vi "test_firmware.vi"() -> ()   [LabVIEW 2025]
panel:
  out "ESP32 Listo":bool
  in  "Close":bool
  out "error out":errorcluster
  in  "stop":bool
  in  "Puerto COM":refnum<visa-resource-name>
  # "Este VI es para comprobar si el firmware fue subido correctamente\nSelecciona el puerto en donde este conectada la ESP32 \nLuego presiona el boton RST de la ESP32\nEspera unos segundos a que este cargue y si todo fue subido correctamente el led se va a encender y la ESP32 ya esta lista para usarse"
  # "Prueba de Firmware"
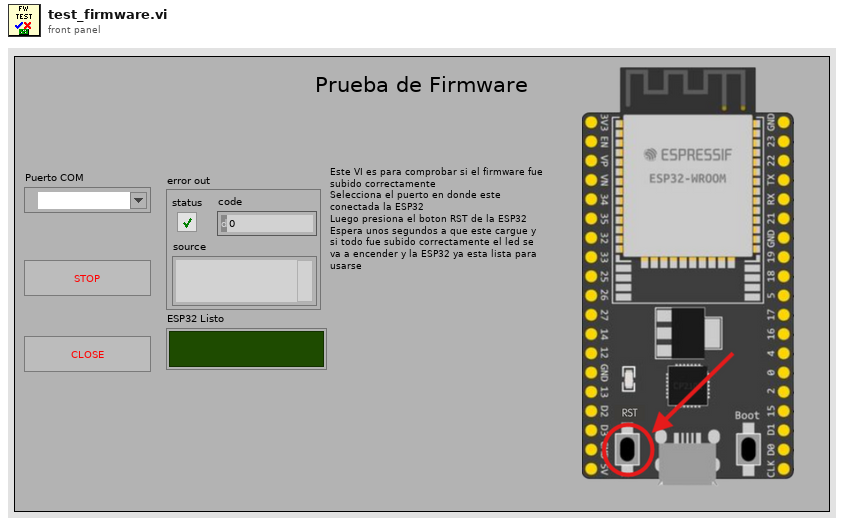
[diagram p1: front panel]
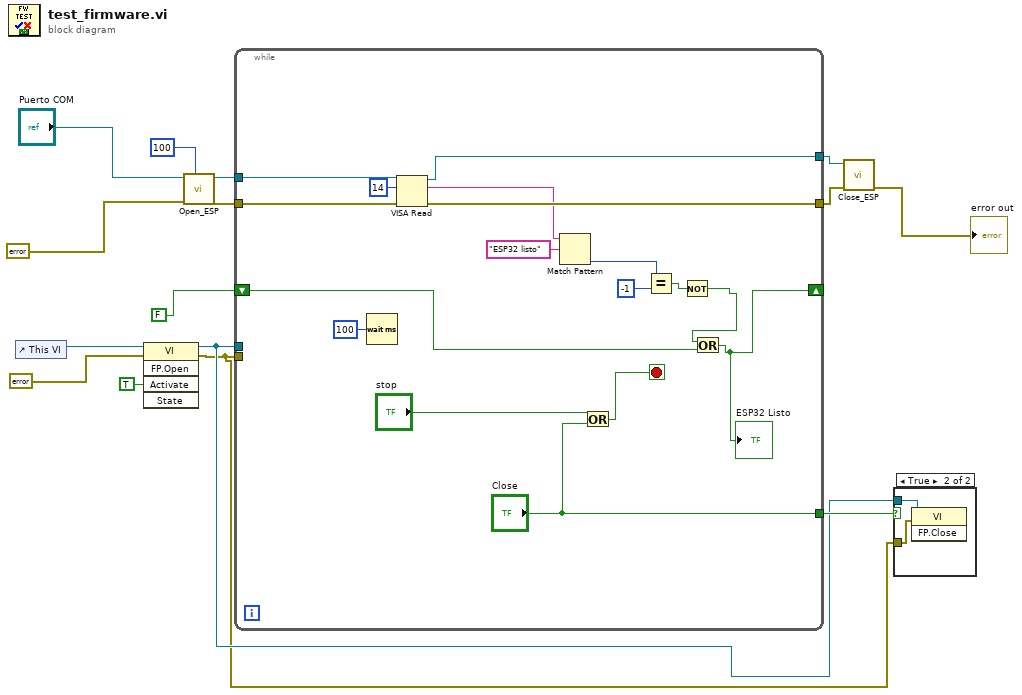
[diagram p0: block diagram]
diagram:
  n1 = control-ref of="This VI"() -> (w9:refnum<vi>)
  n2 = invoke class="VI" method="FP.Open"(reference=w9, error in=errorcluster {"status"=FALSE, "code"=0, "source"=""} ("error in (no error)"), "Activate"=TRUE ("Activate?")) -> (reference out=w3:refnum<vi>, error out=w2:errorcluster)  [unwired: 2 in, 3 out]
  n3 = call "Open_ESP.vi"("timeout (10sec)"=u32 100, "error in (no error)"=errorcluster {"status"=FALSE, "code"=0, "source"=""}, "VISA resource name"="Puerto COM") -> ("error out"=w12:errorcluster, "VISA resource name out"=w15:refnum<visa-resource-name>)  [unwired: 7 in]
  n4 = while {
    tunnel: w15 -> [w29]
    tunnel: [w32] -> w14
    tunnel: [w31] -> w13
    tunnel: w12 -> [w30]
    tunnel: w3 -> [_]
    tunnel: w2 -> [_]
    shift-right: [w16] -> _
    shift-left: FALSE ("Activate?") -> [w20]
    tunnel: ["Close"] -> w4
    stop <- w18 stop-if-true
    n5 = Wait (ms)(milliseconds to wait=u32 100) -> ()  [unwired: 1 out]
    n6 = VISA Read(VISA resource name=w29, byte count=u32 14, error in (no error)=w30) -> (VISA resource name out=w32:refnum<visa-resource-name>, read buffer=w22:string, error out=w31:errorcluster)  [unwired: 1 out]
    n7 = Match Pattern(string=w22, regular expression="ESP32 listo") -> (offset past match=w25:i32)  [unwired: 1 in, 3 out]
    n8 = Or(x="stop", y="Close") -> (x .or. y?=w18:bool)
    n9 = Equal?(x=w25, y=-1) -> (x = y?=w23:bool)
    n10 = Not(x=w23) -> (.not. x?=w21:bool)
    n11 = Or(x=w21, y=w20) -> (x .or. y?=w16:bool)
    "ESP32 Listo" <- w16
  }
  n12 = call "Close_ESP.vi"("error in (no error)"=w13, "VISA resource name"=w14) -> ("error out"=→"error out":errorcluster)  [unwired: 9 in]
  n13 = case shown="True" w4 {
    tunnel: w3 -> [_ w34]
    tunnel: w2 -> [_ w33]
    frame False {
    }
    frame True {
      n14 = invoke class="VI" method="FP.Close"(reference=w34, error in=w33) -> ()  [unwired: 1 in, 3 out]
    }
  }
